vi "Create Waveform.vi"(0 "Sweep Time":dbl format="%#_13g", 2 "Ramp(F)/UpperSine(T)":bool, 5 "Sweep Start Ht":dbl format="%#_13g", 7 "Sweep End Ht":dbl format="%#_13g", 11 "Current Ht":dbl format="%#_13g") -> (4 "Waveform":dbl[](array[numeric]), 8 "Wave.pts":i32, 15 "Current Point":i32)   [LabVIEW 2013]
uses:
  <vilib>/Analysis/1siggen.llb/General Aperiodic Triangle.vi
  <vilib>/Analysis/NI_AALBase.lvlib
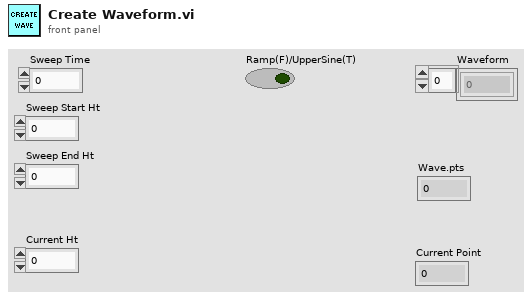
[diagram p1: front panel]
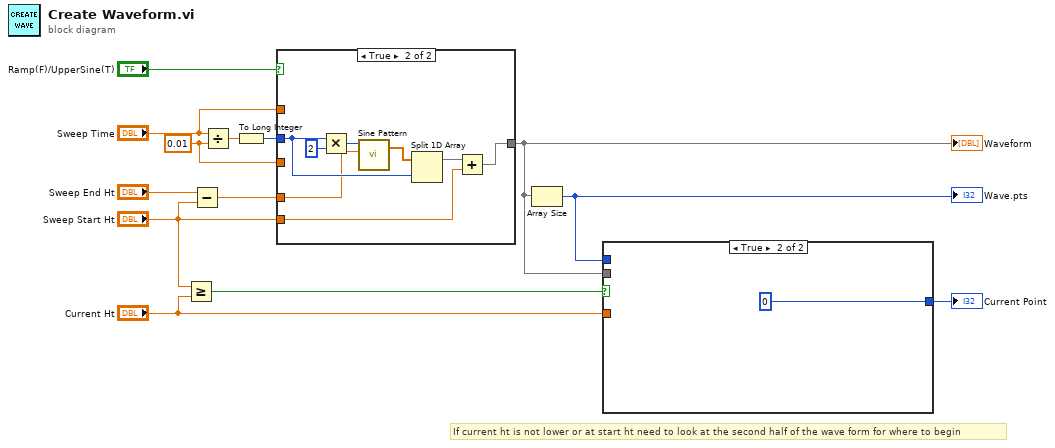
[diagram p0: block diagram]
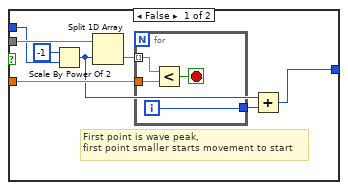
[diagram p2: hidden frame]
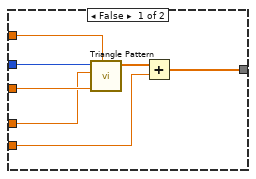
[diagram p3: hidden frame]
diagram:
  w10 = 0.01 ("y")
  # "If current ht is not lower or at start ht need to look at the second half of the wave form for where to begin"
  n1 = Greater Or Equal?(x="Sweep Start Ht", y="Current Ht") -> (x >= y?=w5:bool)
  n2 = Subtract(x="Sweep End Ht", y="Sweep Start Ht") -> (x-y=w7:dbl)
  n3 = Divide(x="Sweep Time", y=w10) -> (x/y=w12:dbl)
  n4 = To Long Integer(number=w12) -> (32bit integer=w11:i32)
  n5 = case shown="True" "Ramp(F)/UpperSine(T)" {
    tunnel: w11 -> [w20 w25]
    tunnel: w10 -> [w19 _]
    tunnel: "Sweep Time" -> [w18 _]
    tunnel: [w14 w21] -> w1
    tunnel: w7 -> [w17 w24]
    tunnel: "Sweep Start Ht" -> [w16 w23]
    frame False {
      n6 = call <vilib>:"Triangle Pattern.vi"("width (s)"=w18, "delta t (s)"=w19, "amplitude"=w17, "samples"=w20) -> ("Triangle Pattern"=w15:dbl[])  [unwired: 6 in, 1 out]
      n7 = Add(x=w15, y=w16) -> (x+y=w14:dbl[])
    }
    frame True {
      n8 = Multiply(x=w25, y=2) -> (x*y=w27:i32)
      n9 = call <vilib>:"Sine Pattern.vi"("amplitude"=w24, "samples"=w27) -> ("Sinusoidal Pattern"=w26:dbl[])  [unwired: 2 in, 1 out]
      n10 = Split 1D Array(array=w26, index=w25) -> (first subarray=w22:dbl[])  [unwired: 1 out]
      n11 = Add(x=w22, y=w23) -> (x+y=w21:dbl[])
    }
  }
  "Waveform" <- w1
  n12 = Array Size(array=w1) -> (size(s)=w3:i32)
  "Wave.pts" <- w3
  n13 = case shown="True" w5 {
    tunnel: "Current Ht" -> [w32 _]
    tunnel: w3 -> [w35 _]
    tunnel: [w29 0] -> w2
    tunnel: w1 -> [w36 _]
    frame False {
      # "First point is wave peak,\nfirst point smaller starts movement to start"
      n14 = Scale By Power Of 2(n=i16 -1, x=w35) -> (x*2^n=w30:i32)
      n15 = Split 1D Array(array=w36, index=w30) -> (second subarray=w33:dbl[])  [unwired: 1 out]
      n16 = for {
        tunnel: w33 -> [w39] mode=indexing
        tunnel: w32 -> [w38]
        tunnel: [w37] -> w31
        i -> [w37]
        stop <- w40 stop-if-true
        n17 = Less?(x=w39, y=w38) -> (x < y?=w40:bool)
      }
      n18 = Add(x=w30, y=w31) -> (x+y=w29:i32)
    }
    frame True {
    }
  }
  "Current Point" <- w2
